vi "reconnect.vi"(8 "error in (no error)":errorcluster, 11 "rethinkdb in":T1) -> (0 "error out":errorcluster, 3 "rethinkdb out":T1)   [LabVIEW 2017, in "rethinkdb.lvlib"]
uses:
  rethinkdb.lvlib
  refnum.ctl
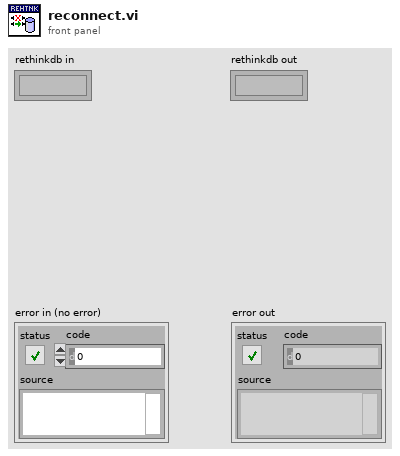
[diagram p1: front panel]
types:
  T1 = typedef "rethinkdb.lvlib/refnum.ctl" = refnum<k1>
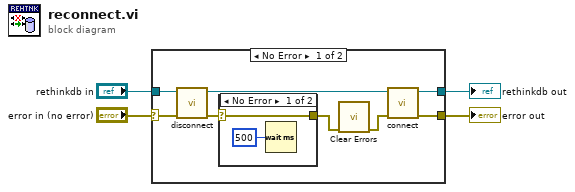
[diagram p0: block diagram]
diagram:
  n1 = case shown="No Error" "error in (no error)" {
    selector: "error in (no error)" -> [w12 w17]
    tunnel: "rethinkdb in" -> [w11 w16]
    tunnel: [w6 w17] -> w3
    tunnel: [w5 w16] -> w1
    frame No Error {
      n2 = call "disconnect.vi"("error in (no error)"=w12, "rethinkdb in"=w11) -> ("error out"=w9:errorcluster, "rethinkdb out"=w10:T1)  [unwired: 8 in]
      n3 = case shown="No Error" w9 {
        selector: w9 -> [w13 w15]
        tunnel: [w13 w15] -> w7
        frame No Error {
          n4 = Wait (ms)(milliseconds to wait=u32 500) -> ()  [unwired: 1 out]
        }
        frame Error {
        }
      }
      n5 = call <vilib>:"Clear Errors.vi"("error in (no error)"=w7) -> ("error out"=w8:errorcluster)  [unwired: 5 in, 1 out]
      n6 = call "connect.vi"("error in (no error)"=w8, "rethinkdb in"=w10) -> ("error out"=w6:errorcluster, "rethinkdb out"=w5:T1)  [unwired: 8 in]
    }
    frame Error {
    }
  }
  "error out" <- w3
  "rethinkdb out" <- w1
